vi "New.vi"(5 "FIFO Options":T2, 7 "fifo depths":u32=10, 8 "error in (no error)":errorcluster, 9 "Logging Interface":refnum<class "Logging Interface.lvclass">, 10 "Thread Parameters":T1={"Priority"=100, "Processor"=-2}, 11 "Plugins":refnum<class "Plugin.lvclass">[](array[class])) -> (0 "error out":errorcluster, 2 "Dispatcher Interface":refnum<class "Dispatcher Interface.lvclass">, 3 "Dispatcher Thread":refnum<class "Dispatcher Thread.lvclass">)   [LabVIEW 2019, in "DSF Core.lvlib" / "Dispatcher Thread.lvclass"]
uses:
  Dispatcher Thread.lvclass
  C:/Dev/GitHub/niveristand-data-sharing-framework-custom-device/Core/Classes/Thread/Thread.lvclass
  Typedefs/DSF FIFO Options.ctl
  Interface/Dispatcher/Dispatcher Interface.lvclass
  C:/Dev/GitHub/niveristand-data-sharing-framework-custom-device/Core/Classes/Interface/Interface.lvclass
  Thread Settings.ctl
  Plugin/Plugin.lvclass
  Interface/Logging/Logging Interface.lvclass
  Interface/Interface.lvclass/Interface.ctl
  Thread.lvclass/Thread.ctl
  Dispatcher Thread.lvclass/Dispatcher Thread.ctl
  Plugin/Plugin.lvclass/Plugin.ctl
  Transfer Group/Transfer Group.lvclass/Transfer Group.ctl
  Interface/New Interface.vi
  Plugin/Get Async Rx Transfer Groups.vi
  Plugin/Get Async Tx Transfer Groups.vi
  Plugin/Get Inline Rx Transfer Groups.vi
  Plugin/Get Inline Tx Transfer Groups.vi
  Transfer Group/Get ID.vi
  Transfer Group/Get Thread.vi
  Plugin/Get Thread Interfaces.vi
  Interface/Create RT FIFO.vi
  Interface/Plugin/Plugin Interface.lvclass
  Thread.lvclass
  Framework/Framework.lvclass
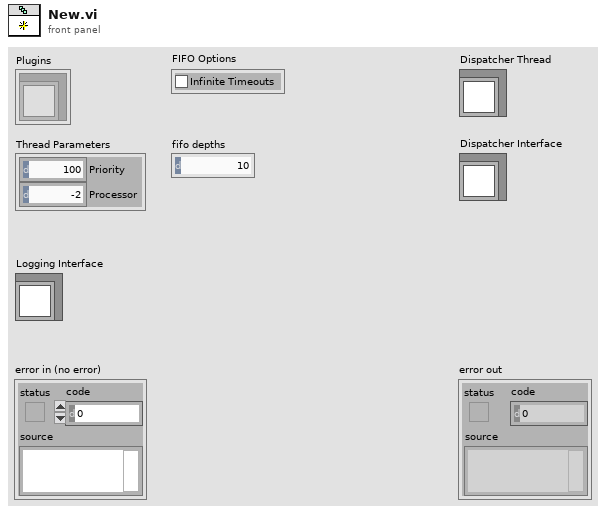
[diagram p1: front panel]
types:
  T1 = typedef "DSF Core.lvlib/Thread.lvclass/Thread Settings.ctl" = cluster{"Priority":u16, "Processor":i32}
  T2 = typedef "DSF Core.lvlib/Framework.lvclass/DSF FIFO Options.ctl" = cluster{"Infinite Timeouts":bool}
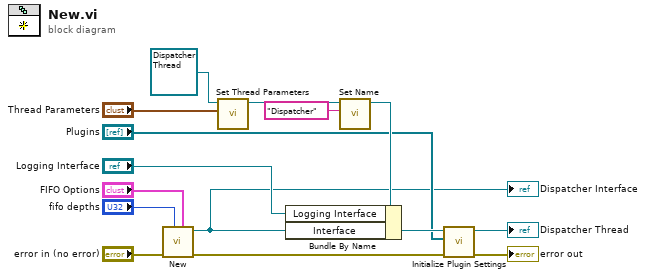
[diagram p0: block diagram]
diagram:
  n1 = call "New.vi"("fifo options"="FIFO Options", "fifo depths (10)"="fifo depths", "error in (no error)"="error in (no error)") -> ("error out"=w5:errorcluster, "Dispatcher Interface"=w3:refnum<class "Dispatcher Interface.lvclass">)  [unwired: 7 in]
  "Dispatcher Interface" <- w3
  n2 = call "Set Thread Parameters.vi"("thread settings"="Thread Parameters", "Thread in"=refnum<class "Dispatcher Thread.lvclass"> refnum ("Dispatcher type")) -> ("Thread out"=w10:refnum<class "Dispatcher Thread.lvclass">)  [unwired: 9 in]
  n3 = call "Set Name.vi"("name"="Dispatcher", "Thread in"=w10) -> ("Thread out"=w9:refnum<class "Dispatcher Thread.lvclass">)  [unwired: 9 in]
  n4 = Bundle By Name(cluster=w9, "Logging Interface"="Logging Interface", "Interface"=w3) -> (w7:refnum<class "Dispatcher Thread.lvclass">)
  n5 = call "Initialize Plugin Settings.vi"("error in (no error)"=w5, "Plugins"="Plugins", "Dispatcher in"=w7) -> ("error out"=→"error out":errorcluster, "Dispatcher out"=→"Dispatcher Thread":refnum<class "Dispatcher Thread.lvclass">)  [unwired: 7 in]
